vi "VelocityTorqueCurrentFOC Setter.vi"(0 "LimitReverseMotion":bool, 1 "FeedForward":dbl, 2 "OverrideCoastDurNeutral":bool, 3 "Update Frequency (Hz)":dbl=100.0, 5 "StopSendingOtherRequests":bool=TRUE, 7 "Velocity":dbl, 9 "Acceleration":dbl, 12 "Slot":i32, 13 "LimitForwardMotion":bool) -> (4 "DeviceReference Out":T1)   [LabVIEW 2023]
doc: "Request PID to target velocity with torque current feedforward.\nThis control mode will set the motor's velocity setpoint to the velocity specified by the user. In addition, it will apply an additional torque current as an arbitrary feedforward value."
uses:
  Users/Cory/Documents/PhoenixPro-LabVIEW-Generation/controls/DeviceReference.ctl
panel:
  in  "DeviceReference":T1
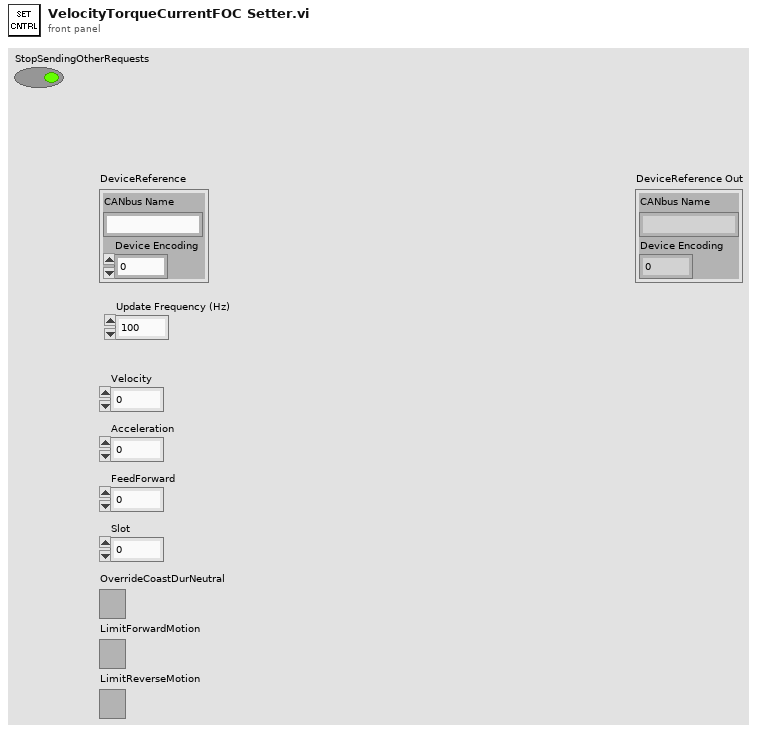
[diagram p1: front panel]
types:
  T1 = typedef "DeviceReference.ctl" = cluster{"CANbus Name":string, "Device Encoding":u32}
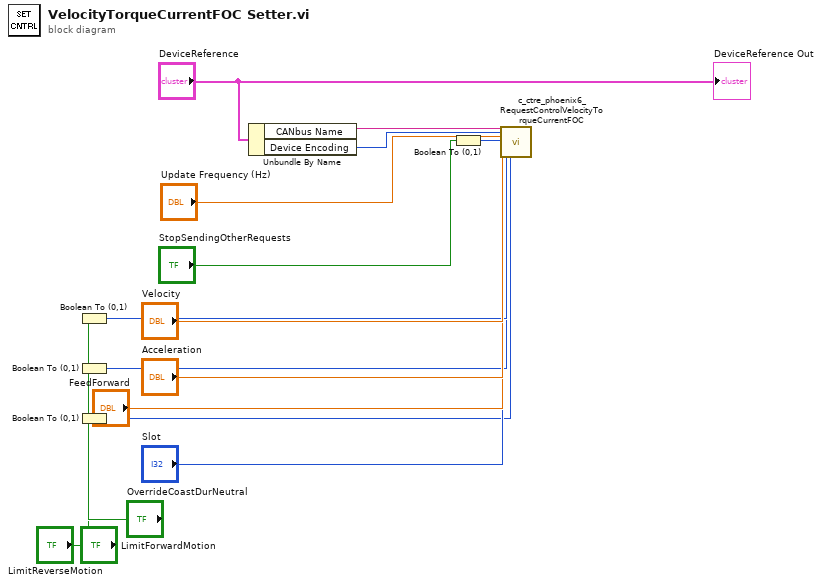
[diagram p0: block diagram]
diagram:
  n1 = Boolean To (0,1)(Boolean="OverrideCoastDurNeutral") -> (0, 1=w5:i16)
  n2 = Boolean To (0,1)(Boolean="LimitForwardMotion") -> (0, 1=w3:i16)
  n3 = Boolean To (0,1)(Boolean="LimitReverseMotion") -> (0, 1=w1:i16)
  n4 = Unbundle By Name("DeviceReference") -> ("CANbus Name"=w15:string, "Device Encoding"=w14:u32)
  n5 = Boolean To (0,1)(Boolean="StopSendingOtherRequests") -> (0, 1=w11:i16)
  n6 = call <vilib>:"c_ctre_phoenix6_RequestControlVelocityTorqueCurrentFOC.vi"("String 2"=w15, "Numeric 2"=w14, "Numeric 3"="Update Frequency (Hz)", "Numeric 4"=w11, "Numeric 5"="Velocity", "Numeric 6"="Acceleration", "Numeric 7"="FeedForward", "Numeric 8"="Slot", "Numeric 9"=w5, "Numeric 10"=w3, "Numeric 11"=w1) -> ()  [unwired: 15 in, 2 out]
  "DeviceReference Out" <- "DeviceReference"
